vi "19-1.vi"() -> ()   [LabVIEW 2019, in "19.lvlib"]
uses:
  19.lvlib
panel:
  in  "Sample?":bool
  out "Number of Beacons":i32
  out "Scanner Orientations Relative to Scanner 0":T1(array[cluster])
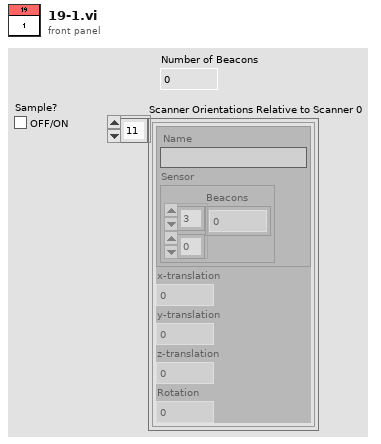
[diagram p1: front panel]
types:
  T1 = cluster{cluster{"Name":string, "Sensor":cluster{"Beacons":i32[][]}}, "x-translation":i32, "y-translation":i32, "z-translation":i32, "Rotation":i32}[]
  T2 = cluster{"Sensor":cluster{"Name":string, "Beacons":i32[][]}, "x Info":cluster{"1st":i32, "12th":i32, "N-12th":i32, "Nth":i32, "Range":i32}, "y Info":cluster{"1st":i32, "12th":i32, "N-12th":i32, "Nth":i32, "Range":i32}, "z Info":cluster{"1st":i32, "12th":i32, "N-12th":i32, "Nth":i32, "Range":i32}}
  T3 = cluster{"Sensor":cluster{"Name":string, "Beacons":i32[][]}, "x Info":cluster{"1st":i32, "12th":i32, "N-12th":i32, "Nth":i32, "Range":i32}, "y Info":cluster{"1st":i32, "12th":i32, "N-12th":i32, "Nth":i32, "Range":i32}, "z Info":cluster{"1st":i32, "12th":i32, "N-12th":i32, "Nth":i32, "Range":i32}}[]
  T4 = cluster{"Sensor":cluster{"Beacons":i32[][]}, "x-translation":i32, "y-translation":i32, "z-translation":i32, "Rotation":i32}
  T5 = cluster{cluster{"Name":string, "Sensor":cluster{"Beacons":i32[][]}}, "x-translation":i32, "y-translation":i32, "z-translation":i32, "Rotation":i32}
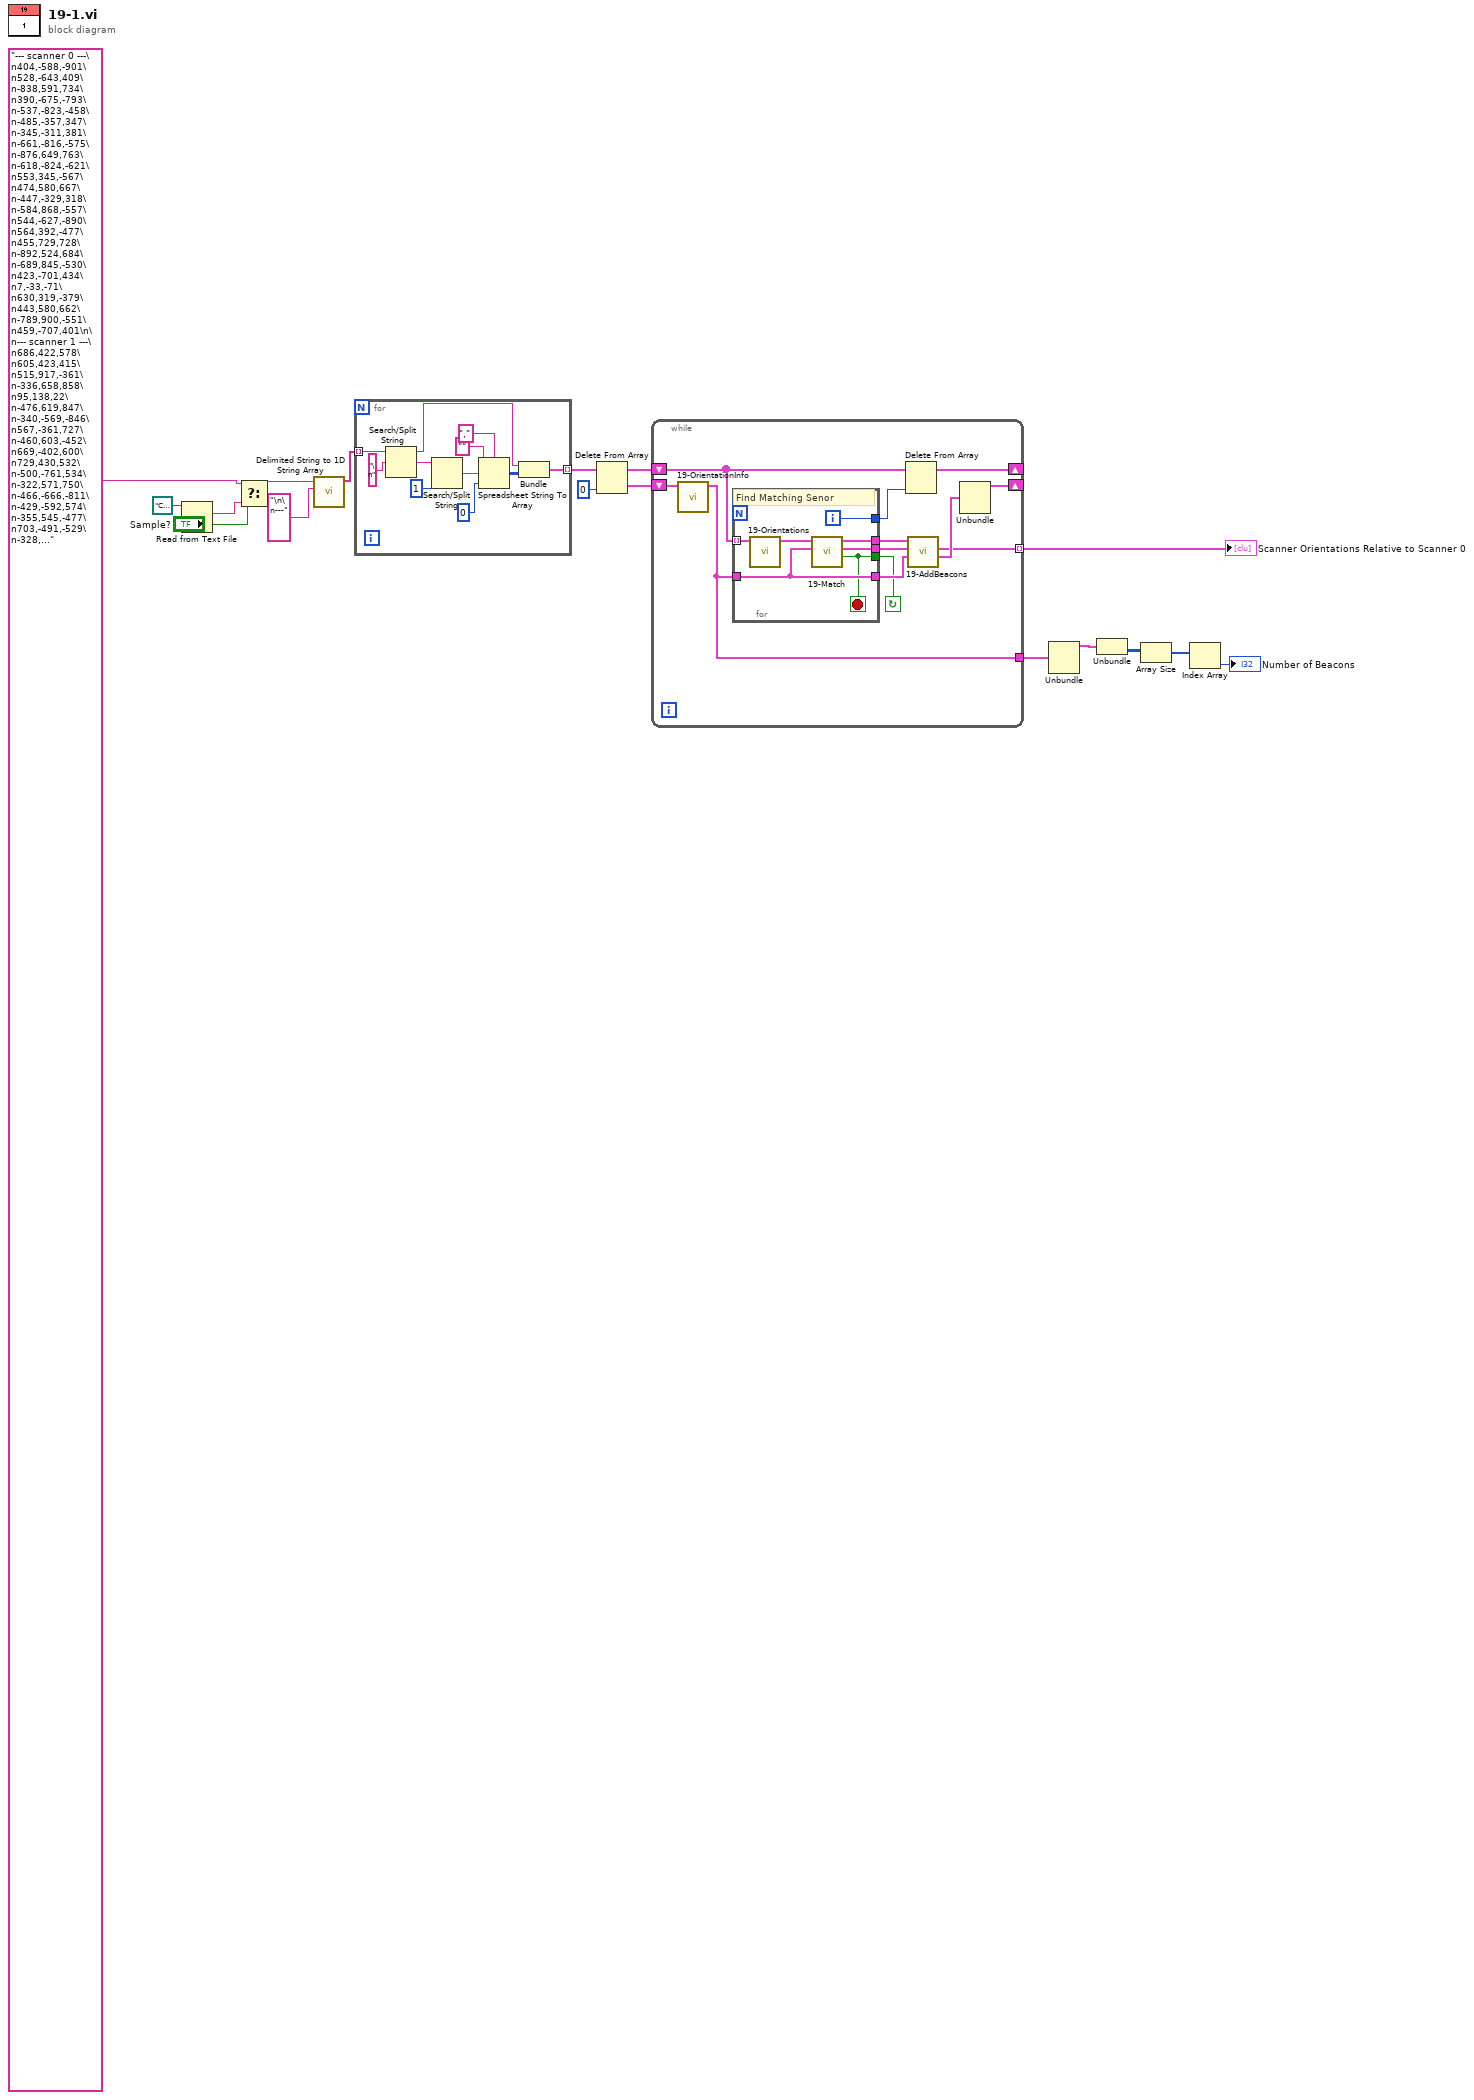
[diagram p0: block diagram]
diagram:
  n1 = Read from Text File(file (use dialog)=path "C:/Users/craig.walker/Documents/GitHub/lv2019-Advent-of-Code-2021/19/input.txt") -> (text=w8:string)  [unwired: 3 in, 3 out]
  n2 = Select(t="--- scanner 0 ---\n404,-588,-901\n528,-643,409\n-838,591,734\n390,-675,-793\n-537,-823,-458\n-485,-357,347\n-345,-311,381\n-661,-816,-575\n-876,649,763\n-618,-824,-621\n553,345,-567\n474,580,667\n-447,-329,318\n-584,868,-557\n544,-627,-890\n564,392,-477\n455,729,728\n-892,524,684\n-689,845,-530\n423,-701,434\n7,-33,-71\n630,319,-379\n443,580,662\n-789,900,-551\n459,-707,401\n\n--- scanner 1 ---\n686,422,578\n605,423,415\n515,917,-361\n-336,658,858\n95,138,22\n-476,619,847\n-340,-569,-846\n567,-361,727\n-460,603,-452\n669,-402,600\n729,430,532\n-500,-761,534\n-322,571,750\n-466,-666,-811\n-429,-592,574\n-355,545,-477\n703,-491,-529\n-328,-685,520\n413,935,-424\n-391,539,-444\n586,-435,557\n-364,-763,-893\n807,-499,-711\n755,-354,-619\n553,889,-390\n\n--- scanner 2 ---\n649,640,665\n682,-795,504\n-784,533,-524\n-644,584,-595\n-588,-843,648\n-30,6,44\n-674,560,763\n500,723,-460\n609,671,-379\n-555,-800,653\n-675,-892,-343\n697,-426,-610\n578,704,681\n493,664,-388\n-671,-858,530\n-667,343,800\n571,-461,-707\n-138,-166,112\n-889,563,-600\n646,-828,498\n640,759,510\n-630,509,768\n-681,-892,-333\n673,-379,-804\n-742,-814,-386\n577,-820,562\n\n--- scanner 3 ---\n-589,542,597\n605,-692,669\n-500,565,-823\n-660,373,557\n-458,-679,-417\n-488,449,543\n-626,468,-788\n338,-750,-386\n528,-832,-391\n562,-778,733\n-938,-730,414\n543,643,-506\n-524,371,-870\n407,773,750\n-104,29,83\n378,-903,-323\n-778,-728,485\n426,699,580\n-438,-605,-362\n-469,-447,-387\n509,732,623\n647,635,-688\n-868,-804,481\n614,-800,639\n595,780,-596\n\n--- scanner 4 ---\n727,592,562\n-293,-554,779\n441,611,-461\n-714,465,-776\n-743,427,-804\n-660,-479,-426\n832,-632,460\n927,-485,-438\n408,393,-506\n466,436,-512\n110,16,151\n-258,-428,682\n-393,719,612\n-211,-452,876\n808,-476,-593\n-575,615,604\n-485,667,467\n-680,325,-822\n-627,-443,-432\n872,-547,-609\n833,512,582\n807,604,487\n839,-516,451\n891,-625,532\n-652,-548,-490\n30,-46,-14", s="Sample?", f=w8) -> (s? t:f=w6:string)
  n3 = call <vilib>:"Delimited String to 1D String Array.vi"("delimiter"="\n\n---", "delimited string"=w6) -> ("string array"=w16:string[])  [unwired: 9 in]
  n4 = for {
    tunnel: w16 -> [w28] mode=indexing
    tunnel: [w20] -> w15 mode=indexing
    n5 = Search/Split String(string=w28, search string/char (-)="\n") -> (substring before match=w18:string, match + rest of string=w27:string)  [unwired: 1 in, 1 out]
    n6 = Search/Split String(string=w27, offset (0)=1) -> (match + rest of string=w25:string)  [unwired: 1 in, 2 out]
    n7 = Spreadsheet String To Array(delimiter (Tab)=",", format string="", spreadsheet string=w25, array type (2D Dbl)=0 ("offset (0)")) -> (array=w19:i32[][])
    n8 = Bundle("String"=w18, w19) -> (w20:cluster{"String":string, i32[][]})  [unwired: 1 in]
  }
  n9 = Delete From Array(array=w15, index=0) -> (deleted portion=w10:cluster{"String":string, i32[][]}, array with subset deleted=w14:cluster{"String":string, i32[][]}[])  [unwired: 1 in]
  n10 = while {
    shift-right: [w38] -> _
    shift-left: w14 -> [w31]
    shift-right: [w39] -> _
    shift-left: w10 -> [w40]
    tunnel: [w33] -> w13 mode=indexing
    tunnel: [w29] -> w3
    stop <- w30 continue-if-true
    n11 = call "19-OrientationInfo.vi"("Sensor in"=w40) -> ("Orientation Info"=w29:T2)  [unwired: 10 in]
    n12 = for {
      tunnel: w31 -> [w46] mode=indexing
      tunnel: [w45] -> w34
      tunnel: w29 -> [w44]
      tunnel: [w44] -> w36
      tunnel: [w43] -> w35
      tunnel: [w42] -> w32
      tunnel: [w41] -> w30
      i -> [w42]
      stop <- w41 stop-if-true
      # "Find Matching Senor"
      n13 = call "19-Orientations.vi"("Sensor"=w46) -> ("Orientations"=w47:T3)  [unwired: 10 in]
      n14 = call "19-Match.vi"("Base Orientation"=w44, "Sensor Orientations"=w47) -> ("Match Found?"=w41:bool, "Match Info"=w43:T4, "Orientation"=w45:T2)  [unwired: 6 in, 1 out]
    }
    n15 = Delete From Array(array=w31, index=w32) -> (array with subset deleted=w38:cluster{"String":string, i32[][]}[])  [unwired: 1 in, 1 out]
    n16 = call "19-AddBeacons.vi"("Base Orientation Info in"=w36, "Match Info"=w35, "Orientation Info in"=w34) -> ("Base Orientation Info out"=w37:T2, "Sensor Match Info"=w33:T5)  [unwired: 7 in]
    n17 = Unbundle(w37) -> ("Sensor"=w39:cluster{"Name":string, "Beacons":i32[][]})  [unwired: 3 out]
  }
  "Scanner Orientations Relative to Scanner 0" <- w13
  n18 = Unbundle(w3) -> ("Sensor"=w2:cluster{"Name":string, "Beacons":i32[][]})  [unwired: 3 out]
  n19 = Unbundle(w2) -> ("Beacons"=w1:i32[][])  [unwired: 1 out]
  n20 = Array Size(array=w1) -> (size(s)=w12:i32[])
  n21 = Index Array(array=w12) -> (element=→"Number of Beacons":i32)  [unwired: 1 in]
